vi "Get Server Internal UEs.vi"(11 "OOP Server in":refnum<class "OOP Query Server.lvclass">) -> (2 "Server Internal UEs":T1, 3 "OOP Server out":refnum<class "OOP Query Server.lvclass">)   [LabVIEW 2019, in "OOP Query Server.lvlib" / "OOP Query Server.lvclass"]
uses:
  OOP Query Server.lvclass
  typeDefs/Server Internal UEs.ctl
  typeDefs/Server Internal Message.ctl
  OOP Query Server.lvclass/OOP Query Server.ctl
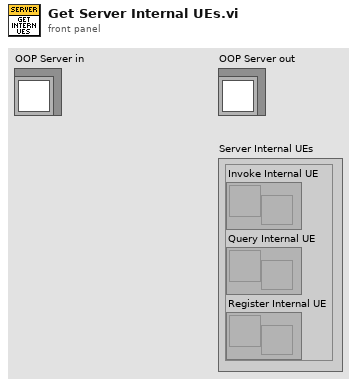
[diagram p1: front panel]
types:
  T1 = typedef "OOP Query Server.lvlib/OOP Query Server.lvclass/Server Internal UEs.ctl" = cluster{"Invoke Internal UE":refnum<user-event>, "Query Internal UE":refnum<user-event>, "Register Internal UE":refnum<user-event>}
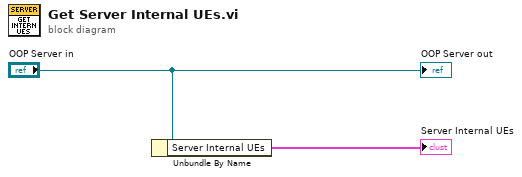
[diagram p0: block diagram]
diagram:
  n1 = Unbundle By Name("OOP Server in") -> ("Server Internal UEs"=→"Server Internal UEs":T1)
  "OOP Server out" <- "OOP Server in"
